vi "Get Auto Config.vi"(11 "Numeric":dbl) -> (3 "Numeric Array":dbl[](array[numeric]))   [LabVIEW 2015]
uses:
  <vilib>/Rock Robotics/Network Tables/NT Read Numeric Array.vi
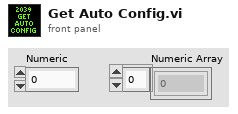
[diagram p1: front panel]
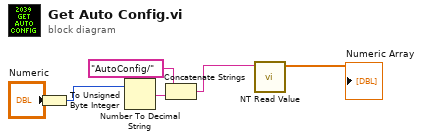
[diagram p0: block diagram]
diagram:
  n1 = To Unsigned Byte Integer(number="Numeric") -> (unsigned 8bit integer=w3:u8)
  n2 = Number To Decimal String(number=w3) -> (decimal integer string=w5:string)  [unwired: 1 in]
  n3 = Concatenate Strings("AutoConfig/", w5) -> (w4:string)
  n4 = call-poly <vilib>:"NT Read Value.vi"("Name"=w4) -> ("Numeric Array"=→"Numeric Array":dbl[])  [unwired: 9 in, 1 out]
